vi "Measurement UI.vi"() -> ()   [LabVIEW 2021, in "Ripple_PMIC.lvlib"]
uses:
  Ripple_PMIC.lvlib
panel:
  in  "Tab Control":enum32{"Ripple Voltage", "Hidden Page"}(tab)
  out "OutputVoltageV/STimeGraph":waveform(dbl)(graph) caption="Ripple"
  in  "Source resource name":string caption="SOURCE DEVICE NAME"
  in  "Load resource name":string caption="LOAD DEVICE NAME"
  in  "Scope resource name":string caption="SCOPE DEVICE NAME"
  out "Source voltage":dbl caption="SOURCE VOLTAGE"
  out "Load current":dbl caption="LOAD CURRENT"
  out "RMS ripple voltage":dbl caption="RMS RIPPLE VOLTAGE"
  out "P-P ripple voltage":dbl caption="P-P RIPPLE VOLTAGE"
  out "Source current":dbl caption="SOURCE CURRENT"
  out "Load voltage":dbl caption="LOAD VOLATGE"
  out "Ripple values":dbl[](array[numeric]) caption="RIPPLE VALUES"
  out "dt":dbl caption="DT"
  out "Results":string[][](table) caption="RESULTS"
  in  "Aperture time":dbl=0.005 caption="APERTURE TIME" format="%#_6ps"
  in  "DUT setup time":dbl=0.005 caption="DUT SETUP TIME" format="%#_6ps"
  in  "Measurement configuration":string="Measurement settings"
  out "Status":string
  in  "Scope probe attenuation":dbl=1.0 caption="PROBE ATTENUATION"
  in  "Source configuration":string="Source configuration"
  in  "Scope configuration":string="Scope configuration"
  in  "Load configuration":string="Load configuration"
  in  "Mode of operation":T1(ring)=enum."Perform measurement" caption="MODE OF OPERATION"
  in  "Scope acquisition time":dbl=3.0 caption="ACQUISTION TIME" format="%#_6ps"
  in  "Scope sample rate":dbl=10000.0 caption="SAMPLE RATE" format="%#_6pHz"
  in  "Scope channel name":string="0" caption="CHANNEL NAME"
  in  "ScopeResourceName":refnum<k15> caption="RESOURCE NAME"
  in  "Load voltage limit range":dbl=6.0 caption="VOLTAGE LIMIT RANGE" format="%#_6pV"
  in  "Load current level":dbl=5.0 caption="CURRENT LEVEL" format="%#_6pA"
  in  "ELOADResourceName":refnum<k15> caption="RESOURCE NAME"
  in  "Source current limit":dbl=15.0 caption="CURRENT LIMIT" format="%#_6pA"
  in  "Source voltage level":dbl=10.0 caption="VOLTAGE LEVEL" format="%#_6pV"
  in  "PPSResourceName":refnum<k15> caption="RESOURCE NAME"
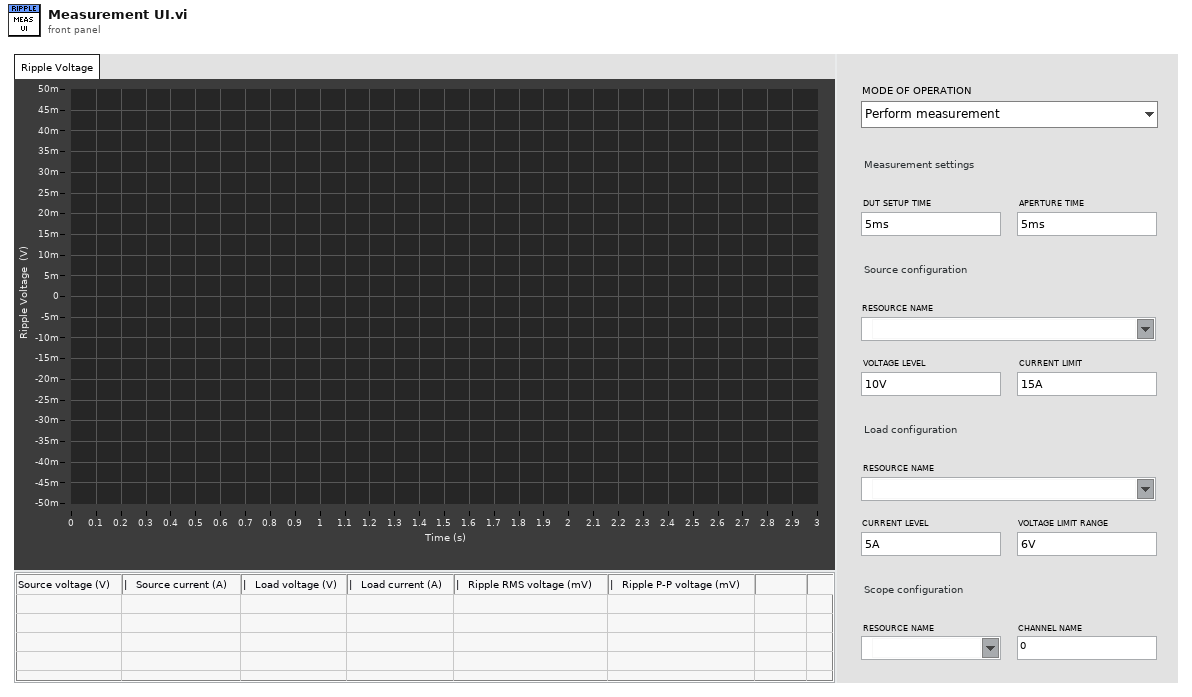
[diagram p1: front panel]
types:
  T1 = enum32{"Power on the DUT", "Perform measurement", "Power off the DUT"}
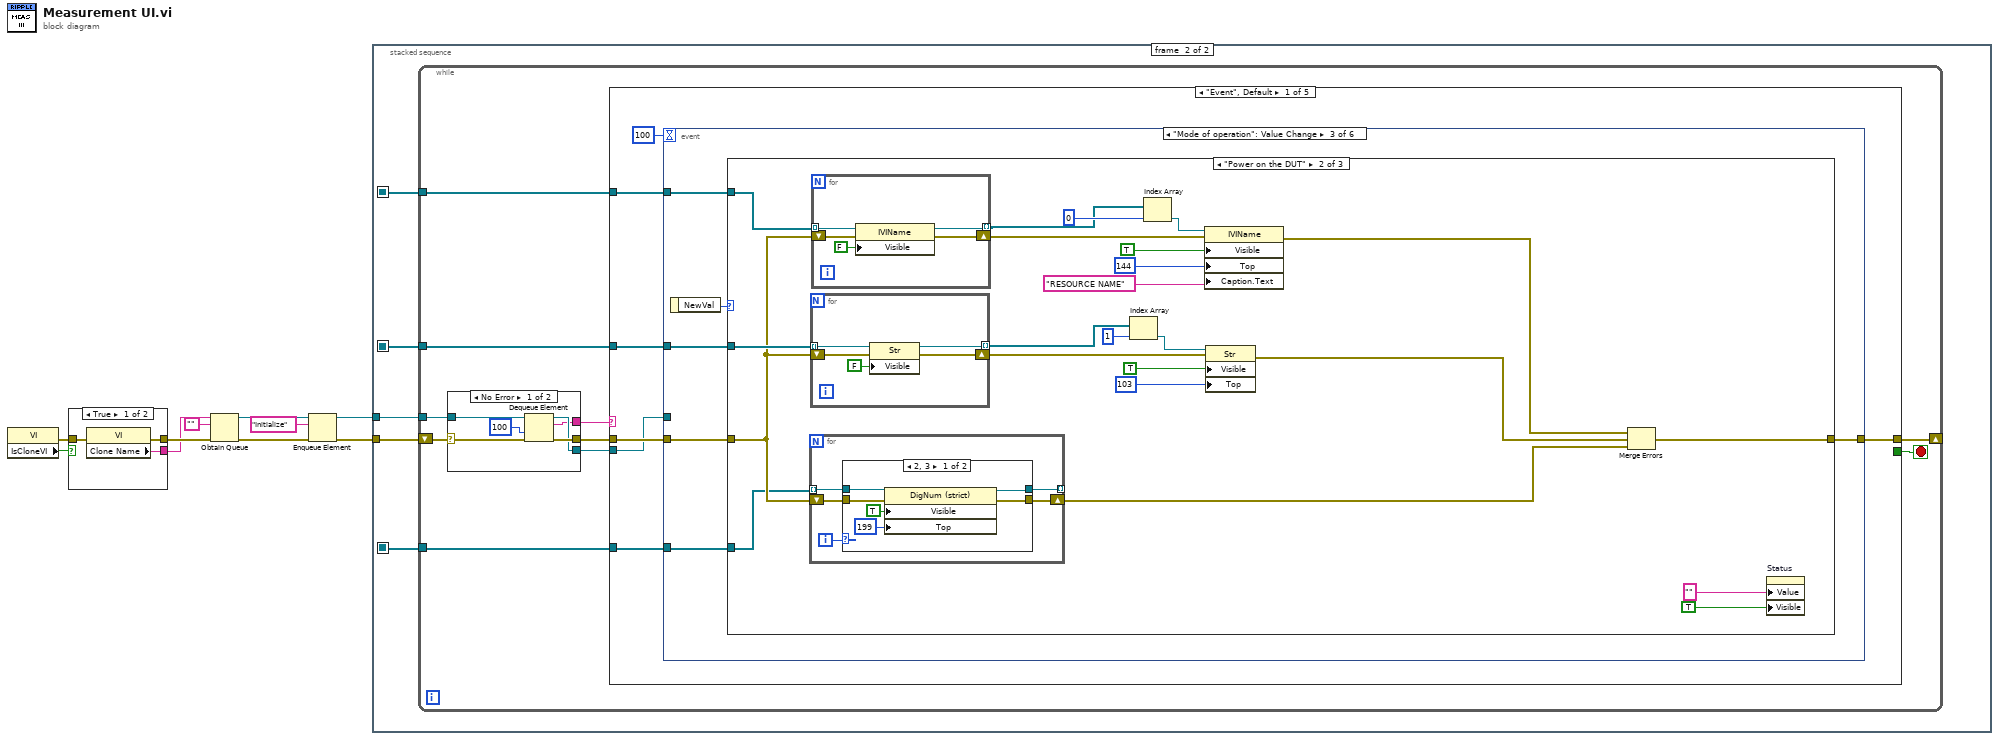
[diagram p0: block diagram]
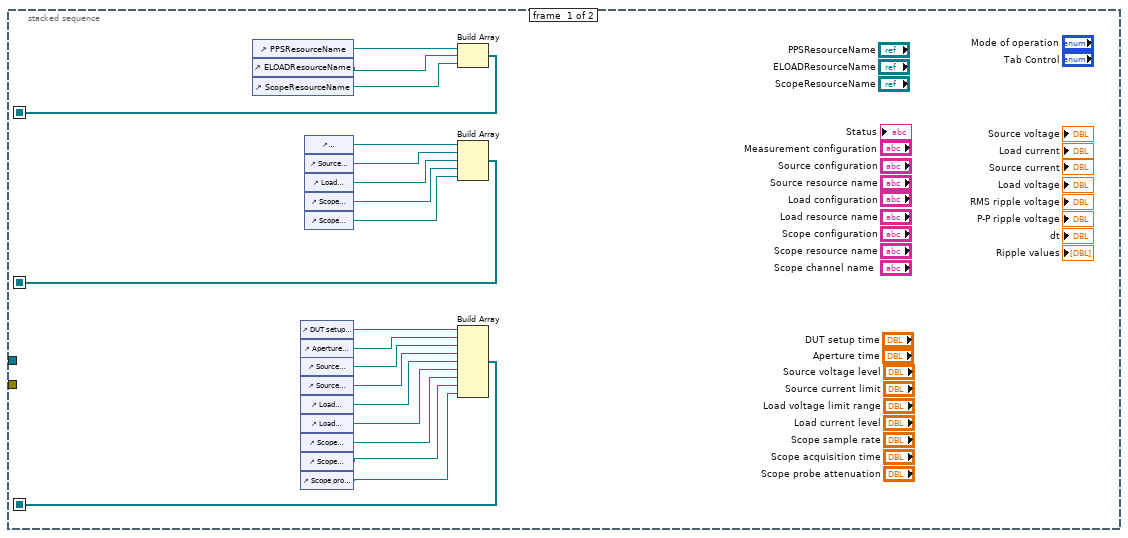
[diagram p2: hidden frame]
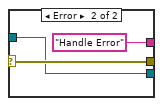
[diagram p3: hidden frame]
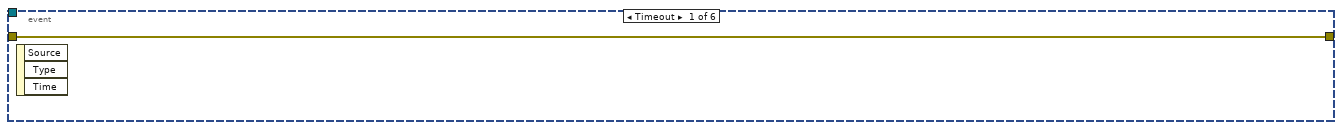
[diagram p4: hidden frame]
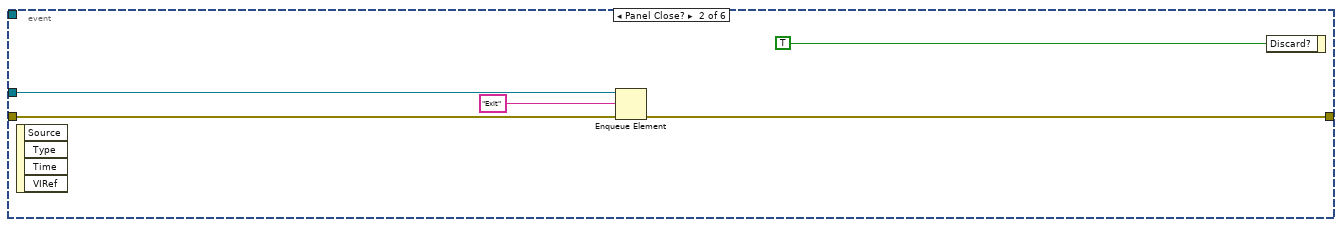
[diagram p5: hidden frame]
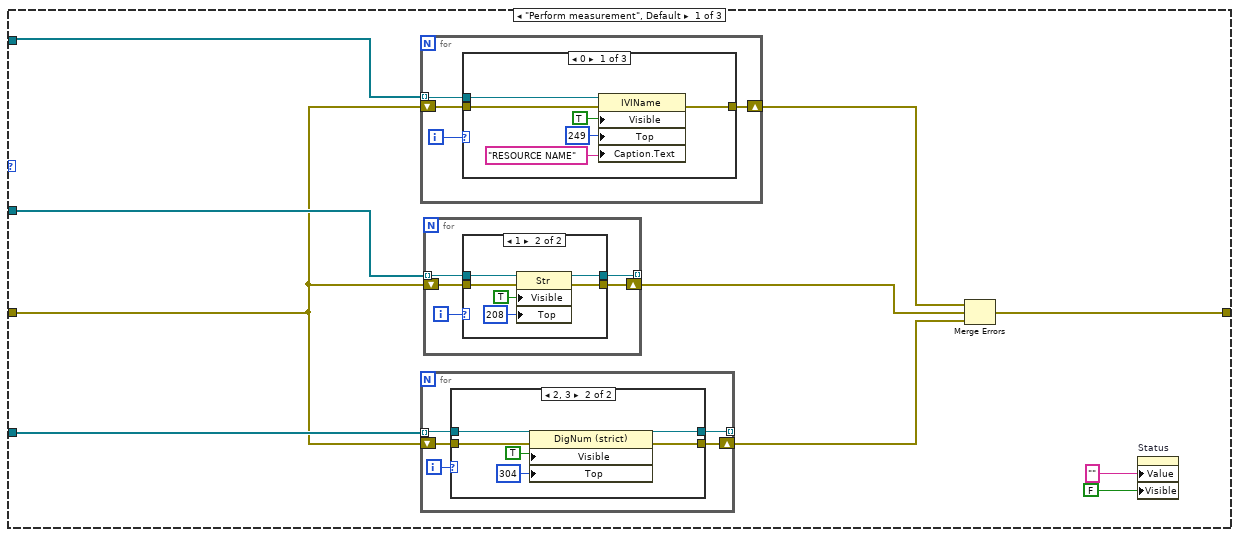
[diagram p6: hidden frame]
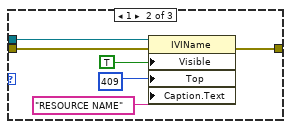
[diagram p7: hidden frame]
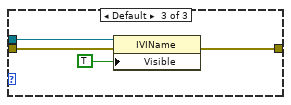
[diagram p8: hidden frame]
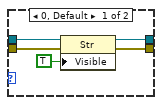
[diagram p9: hidden frame]
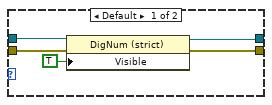
[diagram p10: hidden frame]
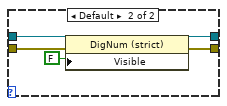
[diagram p11: hidden frame]
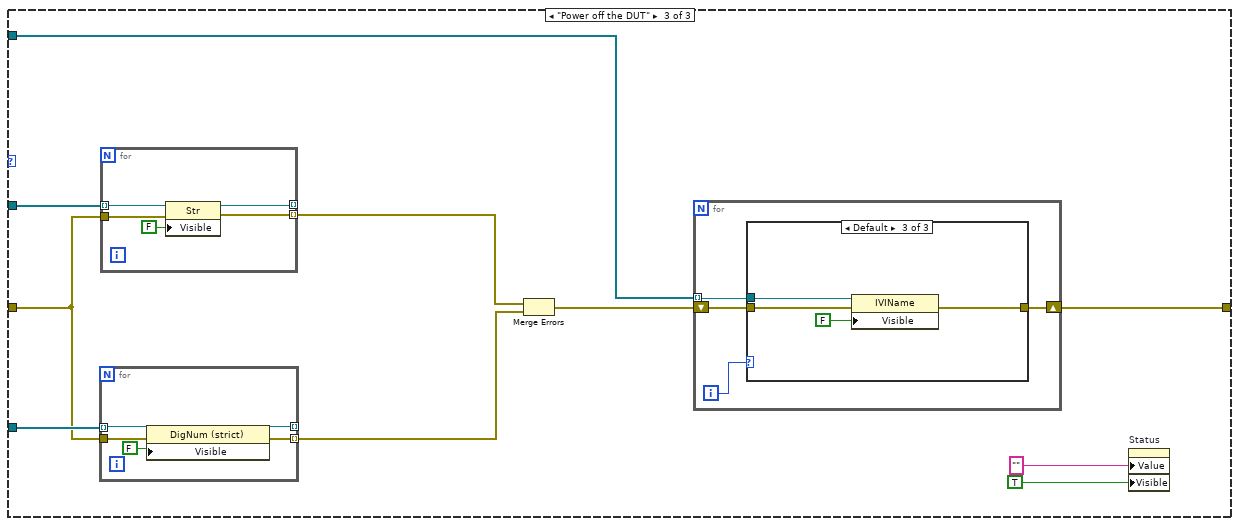
[diagram p12: hidden frame]
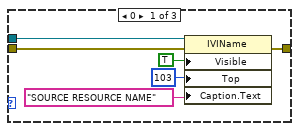
[diagram p13: hidden frame]
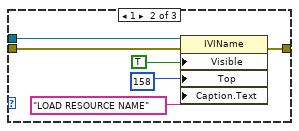
[diagram p14: hidden frame]
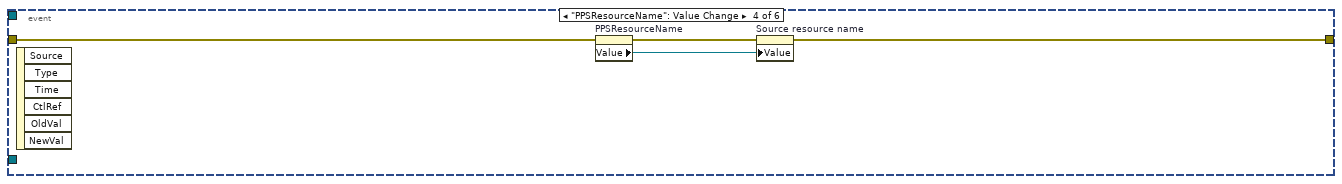
[diagram p15: hidden frame]
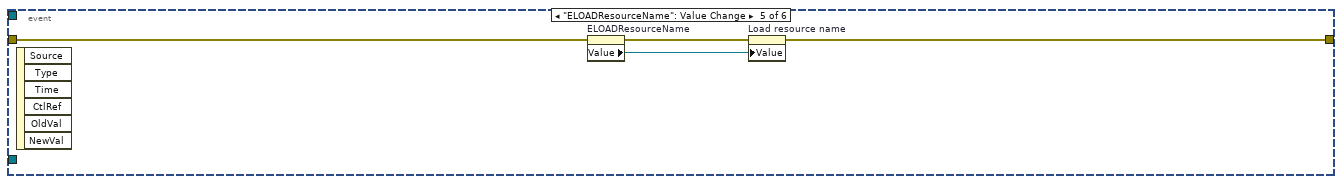
[diagram p16: hidden frame]
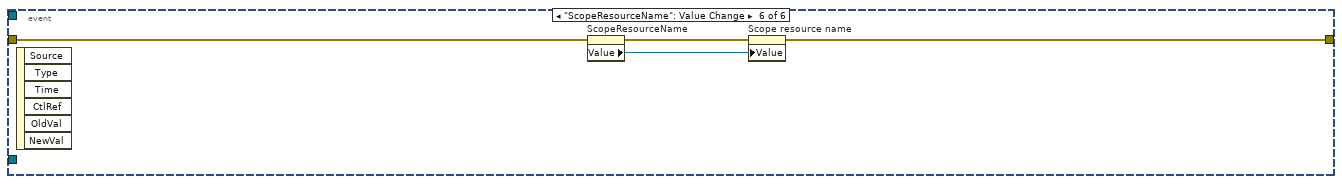
[diagram p17: hidden frame]
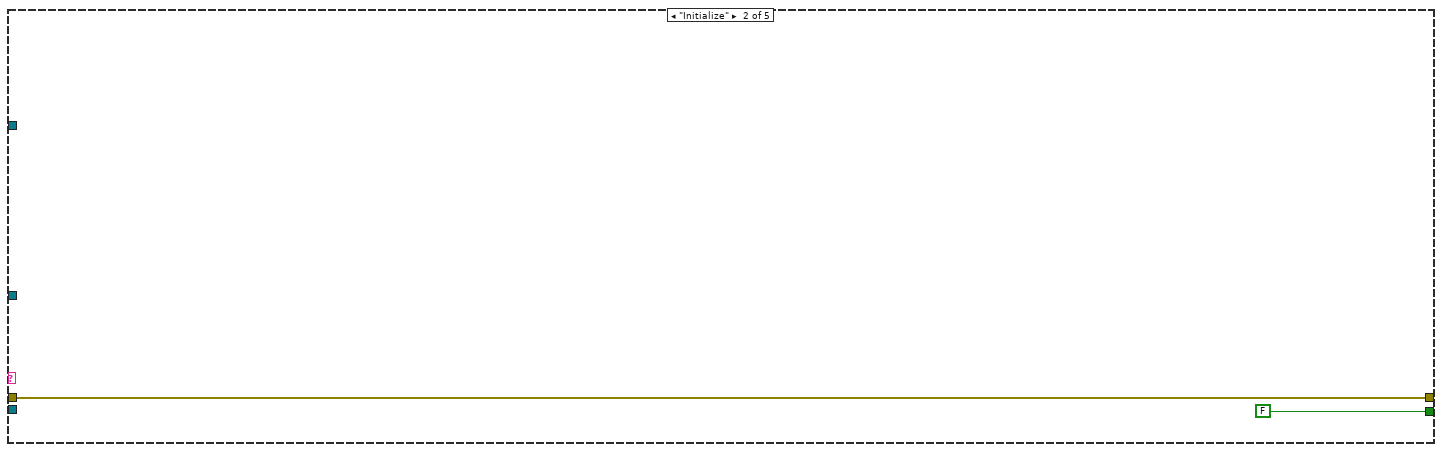
[diagram p18: hidden frame]
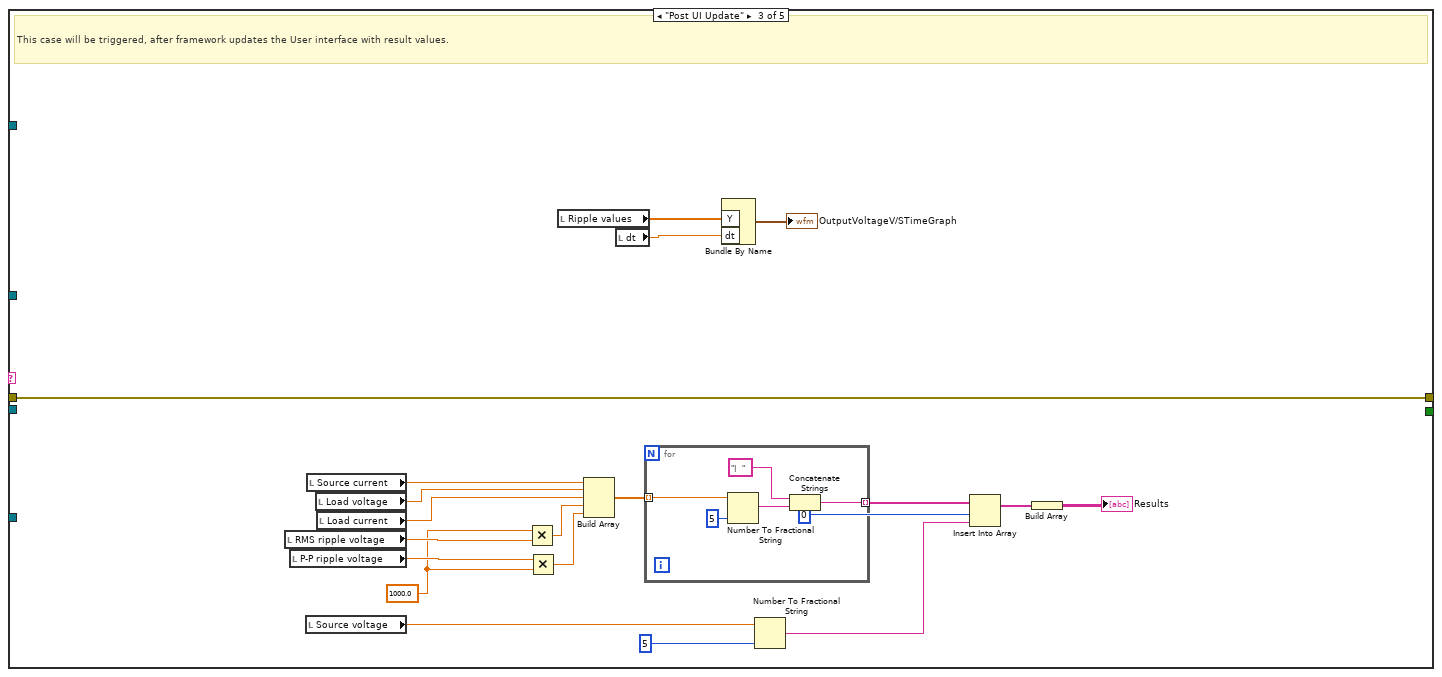
[diagram p19: hidden frame]
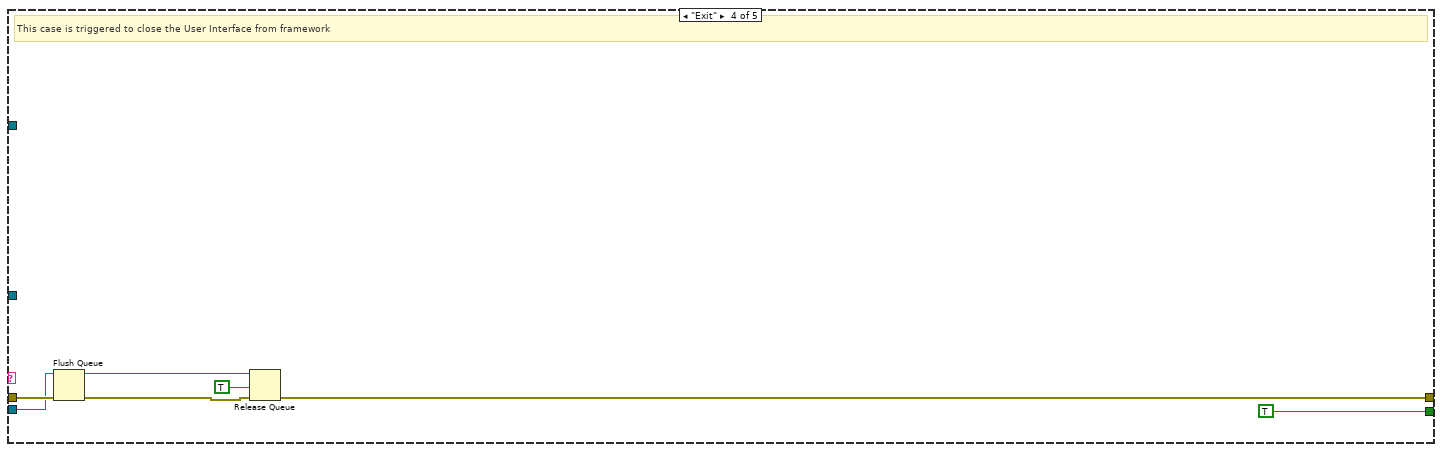
[diagram p20: hidden frame]
diagram:
  n1 = property class="VI"() -> (error out=w1:errorcluster, "IsCloneVI"=w2:bool)  [unwired: 2 in, 1 out]
  n2 = case shown="True" w2 {
    tunnel: [w13 w16] -> w10
    tunnel: [w12 w15] -> w9
    tunnel: w1 -> [w11 w14]
    frame True {
      n3 = property class="VI"(error in=w11) -> (error out=w13:errorcluster, "Clone Name"=w12:string)  [unwired: 1 in, 1 out]
    }
    frame False {
      n4 = property class="VI"(error in=w14) -> (error out=w16:errorcluster, "Name"=w15:string)  [unwired: 1 in, 1 out]
    }
  }
  n5 = Obtain Queue(name (unnamed)=w9, element data type="", error in (no error)=w10) -> (queue out=w6:refnum<queue>, error out=w8:errorcluster)  [unwired: 2 in, 1 out]
  n6 = Enqueue Element(queue=w6, element="Initialize", error in (no error)=w8) -> (queue out=w5:refnum<queue>, error out=w7:errorcluster)  [unwired: 1 in, 1 out]
  n7 = stacked-sequence {
    seq-local: [w25 _] -> [_ w37]
    seq-local: [w24 _] -> [_ w39]
    seq-local: [w23 _] -> [_ w38]
    tunnel: w7 -> [_ w41]
    tunnel: w5 -> [_ w40]
    frame #0 {
      n8 = control-ref of="PPSResourceName"() -> (w28:refnum<vi>)
      n9 = control-ref of="ELOADResourceName"() -> (w27:refnum<vi>)
      n10 = control-ref of="ScopeResourceName"() -> (w26:refnum<vi>)
      n11 = control-ref of="DUT setup time"() -> (w18:refnum<vi>)
      n12 = control-ref of="Aperture time"() -> (w17:refnum<vi>)
      n13 = control-ref of="Source voltage level"() -> (w36:refnum<vi>)
      n14 = control-ref of="Source current limit"() -> (w34:refnum<vi>)
      n15 = control-ref of="Load voltage limit range"() -> (w32:refnum<vi>)
      n16 = control-ref of="Load current level"() -> (w31:refnum<vi>)
      n17 = control-ref of="Scope sample rate"() -> (w30:refnum<vi>)
      n18 = control-ref of="Scope acquisition time"() -> (w33:refnum<vi>)
      n19 = control-ref of="Scope probe attenuation"() -> (w35:refnum<vi>)
      n20 = control-ref of="Measurement configuration"() -> (w19:refnum<vi>)
      n21 = control-ref of="Source configuration"() -> (w29:refnum<vi>)
      n22 = control-ref of="Load configuration"() -> (w22:refnum<vi>)
      n23 = control-ref of="Scope configuration"() -> (w21:refnum<vi>)
      n24 = control-ref of="Scope channel name"() -> (w20:refnum<vi>)
      n25 = Build Array(w28, w27, w26) -> (w25:refnum<vi>[])
      n26 = Build Array(w19, w29, w22, w21, w20) -> (w24:refnum<vi>[])
      n27 = Build Array(w18, w17, w36, w34, w32, w31, w30, w33, w35) -> (w23:refnum<vi>[])
    }
    frame #1 {
      n28 = while {
        shift-right: [w46] -> _
        shift-left: w41 -> [w51]
        tunnel: w40 -> [w49]
        tunnel: w39 -> [w44]
        tunnel: w38 -> [w43]
        tunnel: w37 -> [w42]
        stop <- w45 stop-if-true
        n29 = case shown="No Error" w51 {
          selector: w51 -> [w57 w60]
          tunnel: [w56 w60] -> w50
          tunnel: w49 -> [w55 w59]
          tunnel: [w54 w59] -> w48
          tunnel: [w53 "Handle Error"] -> w47
          frame No Error {
            n30 = Dequeue Element(queue=w55, timeout in ms (-1)=100, error in (no error)=w57) -> (queue out=w54:refnum<queue>, element=w53:string, error out=w56:errorcluster)  [unwired: 1 out]
          }
          frame Error {
          }
        }
        n31 = case shown="\"Event\", Default" w47 {
          tunnel: w50 -> [w66 w243 w250 w276 w277]
          tunnel: w48 -> [w65 _ _ w274 _]
          tunnel: [w67 w243 w250 w271 w277] -> w46
          tunnel: [_ FALSE _ TRUE _] -> w45
          tunnel: w44 -> [w63 _ _ _ _]
          tunnel: w43 -> [w62 _ _ _ _]
          tunnel: w42 -> [w61 _ _ _ _]
          frame "Event", Default {
            n32 = event shown="[2] \"Mode of operation\": Value Change" {
              selector: _ -> [_ _ _ _ _ _]
              dyn-events: _ -> [_ _ _ _ _ _]
              timeout: 100 -> [_ _ _ _ _ _]
              tunnel: [w68 w72 w74 w231 w235 w239] -> w67
              tunnel: w66 -> [w68 w73 w79 w233 w237 w241]
              tunnel: w65 -> [_ w71 _ _ _ _]
              tunnel: w63 -> [_ _ w77 _ _ _]
              tunnel: w62 -> [_ _ w76 _ _ _]
              tunnel: w61 -> [_ _ w75 _ _ _]
              event Timeout {
                n33 = event-data() -> ()  [unwired: 1 in, 3 out]
              }
              event Panel Close? {
                n34 = event-data() -> ()  [unwired: 1 in, 4 out]
                n35 = Enqueue Element(queue=w71, element="Exit", error in (no error)=w73) -> (error out=w72:errorcluster)  [unwired: 1 in, 2 out]
                n36 = event-data("Discard?"=TRUE) -> ()  [unwired: 1 in, 1 out]
              }
              event "Mode of operation": Value Change {
                n37 = event-data() -> ("NewVal"=w78:T1)  [unwired: 1 in]
                n38 = case shown="\"Power on the DUT\"" w78 {
                  tunnel: w79 -> [w84 w157 w198]
                  tunnel: w77 -> [w89 w164 w199]
                  tunnel: w76 -> [w88 w156 w200]
                  tunnel: w75 -> [w87 w158 w197]
                  tunnel: [w83 w146 w193] -> w74
                  frame "Perform measurement", Default {
                    n39 = for {
                      shift-right: [w91] -> w82
                      shift-left: w84 -> [w92]
                      tunnel: w87 -> [w90] mode=indexing
                      i -> [w93]
                      n40 = case shown="0" w93 {
                        tunnel: w92 -> [w96 w102 w109]
                        tunnel: [w95 w101 w107] -> w91
                        tunnel: w90 -> [w94 w100 w106]
                        frame 0 {
                          n41 = property class="IVIName"(reference=w94, error in=w96, "Visible"=TRUE, "Top"=249 ("Position:Top"), "Caption.Text"="RESOURCE NAME") -> (error out=w95:errorcluster)  [unwired: 1 out]
                        }
                        frame 1 {
                          n42 = property class="IVIName"(reference=w100, error in=w102, "Visible"=TRUE, "Top"=409 ("Position:Top"), "Caption.Text"="RESOURCE NAME") -> (error out=w101:errorcluster)  [unwired: 1 out]
                        }
                        frame Default {
                          n43 = property class="IVIName"(reference=w106, error in=w109, "Visible"=TRUE) -> (error out=w107:errorcluster)  [unwired: 1 out]
                        }
                      }
                    }
                    n44 = for {
                      tunnel: w88 -> [w130] mode=indexing
                      tunnel: [w129] -> _ mode=indexing
                      shift-right: [w127] -> w80
                      shift-left: w84 -> [w128]
                      i -> [w126]
                      n45 = case shown="2, 3" w126 {
                        tunnel: w130 -> [w135 w141]
                        tunnel: [w132 w139] -> w129
                        tunnel: w128 -> [w134 w138]
                        tunnel: [w133 w137] -> w127
                        frame Default {
                          n46 = property class="DigNum (strict)"(reference=w135, error in=w134, "Visible"=TRUE) -> (reference out=w132:refnum<vi>, error out=w133:errorcluster)
                        }
                        frame 2, 3 {
                          n47 = property class="DigNum (strict)"(reference=w141, error in=w138, "Visible"=TRUE, "Top"=304 ("Position:Top")) -> (reference out=w139:refnum<vi>, error out=w137:errorcluster)
                        }
                      }
                    }
                    n48 = for {
                      tunnel: w89 -> [w114] mode=indexing
                      tunnel: [w112] -> _ mode=indexing
                      shift-right: [w111] -> w81
                      shift-left: w84 -> [w113]
                      i -> [w110]
                      n49 = case shown="1" w110 {
                        tunnel: w114 -> [w118 w124]
                        tunnel: w113 -> [w115 w123]
                        tunnel: [w117 w122] -> w112
                        tunnel: [w116 w121] -> w111
                        frame 0, Default {
                          n50 = property class="Str"(reference=w118, error in=w115, "Visible"=TRUE) -> (reference out=w117:refnum<vi>, error out=w116:errorcluster)
                        }
                        frame 1 {
                          n51 = property class="Str"(reference=w124, error in=w123, "Visible"=TRUE, "Top"=208 ("Position:Top")) -> (reference out=w122:refnum<vi>, error out=w121:errorcluster)
                        }
                      }
                    }
                    n52 = Merge Errors(w82, w81, w80) -> (w83:errorcluster)
                    n53 = property on="Status" class="Str"("Value"="" ("Status"), "Visible"=FALSE) -> ()  [unwired: 2 in, 2 out]
                  }
                  frame "Power on the DUT" {
                    n54 = for {
                      tunnel: w156 -> [w179] mode=indexing
                      tunnel: [w178] -> _ mode=indexing
                      shift-right: [w176] -> w142
                      shift-left: w157 -> [w177]
                      i -> [w175]
                      n55 = case shown="2, 3" w175 {
                        tunnel: w179 -> [w183 w190]
                        tunnel: [w185 w188] -> w178
                        tunnel: w177 -> [w182 w187]
                        tunnel: [w184 w186] -> w176
                        frame 2, 3 {
                          n56 = property class="DigNum (strict)"(reference=w183, error in=w182, "Visible"=TRUE, "Top"=199 ("Position:Top")) -> (reference out=w185:refnum<vi>, error out=w184:errorcluster)
                        }
                        frame Default {
                          n57 = property class="DigNum (strict)"(reference=w190, error in=w187, "Visible"=FALSE) -> (reference out=w188:refnum<vi>, error out=w186:errorcluster)
                        }
                      }
                    }
                    n58 = for {
                      tunnel: w164 -> [w173] mode=indexing
                      tunnel: [w171] -> w160 mode=indexing
                      shift-right: [w170] -> w161
                      shift-left: w157 -> [w172]
                      n59 = property class="Str"(reference=w173, error in=w172, "Visible"=FALSE) -> (reference out=w171:refnum<vi>, error out=w170:errorcluster)
                    }
                    n60 = for {
                      tunnel: w158 -> [w168] mode=indexing
                      tunnel: [w166] -> w151 mode=indexing
                      shift-right: [w165] -> w152
                      shift-left: w157 -> [w167]
                      n61 = property class="IVIName"(reference=w168, error in=w167, "Visible"=FALSE) -> (reference out=w166:refnum<vi>, error out=w165:errorcluster)
                    }
                    n62 = Index Array(array=w160, index=1) -> (element=w159:refnum<vi>)
                    n63 = Index Array(array=w151, index=0) -> (element=w153:refnum<vi>)
                    n64 = property class="IVIName"(reference=w153, error in=w152, "Visible"=TRUE, "Top"=144 ("Position:Top"), "Caption.Text"="RESOURCE NAME") -> (error out=w147:errorcluster)  [unwired: 1 out]
                    n65 = property class="Str"(reference=w159, error in=w161, "Visible"=TRUE, "Top"=103 ("Position:Top")) -> (error out=w148:errorcluster)  [unwired: 1 out]
                    n66 = Merge Errors(w147, w148, w142) -> (w146:errorcluster)
                    n67 = property on="Status" class="Str"("Value"="" ("Status"), "Visible"=TRUE) -> ()  [unwired: 2 in, 2 out]
                  }
                  frame "Power off the DUT" {
                    n68 = for {
                      tunnel: w200 -> [w230] mode=indexing
                      tunnel: [w228] -> _ mode=indexing
                      tunnel: w198 -> [w227]
                      tunnel: [w226] -> w195 mode=indexing
                      n69 = property class="DigNum (strict)"(reference=w230, error in=w227, "Visible"=FALSE) -> (reference out=w228:refnum<vi>, error out=w226:errorcluster)
                    }
                    n70 = for {
                      tunnel: w199 -> [w224] mode=indexing
                      tunnel: w198 -> [w223]
                      tunnel: [w222] -> _ mode=indexing
                      tunnel: [w221] -> w196 mode=indexing
                      n71 = property class="Str"(reference=w224, error in=w223, "Visible"=FALSE) -> (reference out=w222:refnum<vi>, error out=w221:errorcluster)
                    }
                    n72 = Merge Errors(w196, w195) -> (w194:errorcluster)
                    n73 = for {
                      tunnel: w197 -> [w203] mode=indexing
                      shift-right: [w201] -> w193
                      shift-left: w194 -> [w202]
                      i -> [w204]
                      n74 = case shown="Default" w204 {
                        tunnel: w203 -> [w207 w212 w220]
                        tunnel: w202 -> [w206 w213 w219]
                        tunnel: [w205 w211 w217] -> w201
                        frame 0 {
                          n75 = property class="IVIName"(reference=w207, error in=w206, "Visible"=TRUE, "Top"=103 ("Position:Top"), "Caption.Text"="SOURCE RESOURCE NAME") -> (error out=w205:errorcluster)  [unwired: 1 out]
                        }
                        frame 1 {
                          n76 = property class="IVIName"(reference=w212, error in=w213, "Visible"=TRUE, "Top"=158 ("Position:Top"), "Caption.Text"="LOAD RESOURCE NAME") -> (error out=w211:errorcluster)  [unwired: 1 out]
                        }
                        frame Default {
                          n77 = property class="IVIName"(reference=w220, error in=w219, "Visible"=FALSE) -> (error out=w217:errorcluster)  [unwired: 1 out]
                        }
                      }
                    }
                    n78 = property on="Status" class="Str"("Value"="" ("Status"), "Visible"=TRUE) -> ()  [unwired: 2 in, 2 out]
                  }
                }
              }
              event "PPSResourceName": Value Change {
                n79 = event-data() -> ()  [unwired: 1 in, 6 out]
                n80 = property on="PPSResourceName" class="IVIName"(error in=w233) -> (error out=w232:errorcluster, "Value"=w234:refnum<k15>)  [unwired: 1 in, 1 out]
                n81 = property on="Source resource name" class="Str"(error in=w232, "Value"=w234) -> (error out=w231:errorcluster)  [unwired: 1 in, 1 out]
              }
              event "ELOADResourceName": Value Change {
                n82 = event-data() -> ()  [unwired: 1 in, 6 out]
                n83 = property on="ELOADResourceName" class="IVIName"(error in=w237) -> (error out=w236:errorcluster, "Value"=w238:refnum<k15>)  [unwired: 1 in, 1 out]
                n84 = property on="Load resource name" class="Str"(error in=w236, "Value"=w238) -> (error out=w235:errorcluster)  [unwired: 1 in, 1 out]
              }
              event "ScopeResourceName": Value Change {
                n85 = event-data() -> ()  [unwired: 1 in, 6 out]
                n86 = property on="ScopeResourceName" class="IVIName"(error in=w241) -> (error out=w240:errorcluster, "Value"=w242:refnum<k15>)  [unwired: 1 in, 1 out]
                n87 = property on="Scope resource name" class="Str"(error in=w240, "Value"=w242) -> (error out=w239:errorcluster)  [unwired: 1 in, 1 out]
              }
            }
          }
          frame "Initialize" {
          }
          frame "Post UI Update" {
            w247 = 1000.0 ("x")
            # "This case will be triggered, after framework updates the User interface with result values."
            n88 = local read "RMS ripple voltage"() -> (w248:dbl)
            n89 = local read "P-P ripple voltage"() -> (w249:dbl)
            n90 = local read "Source voltage"() -> (w256:dbl)
            n91 = local read "Source current"() -> (w261:dbl)
            n92 = local read "Load voltage"() -> (w260:dbl)
            n93 = local read "Load current"() -> (w259:dbl)
            n94 = Multiply(x=w247, y=w248) -> (x*y=w246:dbl)
            n95 = Multiply(x=w249, y=w247) -> (x*y=w245:dbl)
            n96 = local read "Ripple values"() -> (w264:dbl[])
            n97 = Build Array(w261, w260, w259, w246, w245) -> (w258:dbl[])
            n98 = local read "dt"() -> (w263:dbl)
            n99 = for {
              tunnel: w258 -> [w268] mode=indexing
              tunnel: [w265] -> w255 mode=indexing
              n100 = Number To Fractional String(number=w268, precision (6)=i16 5) -> (F-format string=w267:string)  [unwired: 2 in]
              n101 = Concatenate Strings("|   " ("string"), w267) -> (w265:string)
            }
            n102 = Bundle By Name("Y"=w264, "dt"=w263) -> (→"OutputVoltageV/STimeGraph":waveform(dbl))  [unwired: 1 in]
            n103 = Number To Fractional String(number=w256, precision (6)=i16 5) -> (F-format string=w254:string)  [unwired: 2 in]
            n104 = Insert Into Array(array=w255, index=0, new element=w254) -> (w252:string[])
            n105 = Build Array(w252) -> (→"Results":string[][])
          }
          frame "Exit" {
            # "This case is triggered to close the User Interface from framework"
            n106 = Flush Queue(queue=w274, error in (no error)=w276) -> (queue out=w273:refnum<queue>, error out=w272:errorcluster)  [unwired: 1 out]
            n107 = Release Queue(queue=w273, force destroy? (F)=TRUE, error in (no error)=w272) -> (error out=w271:errorcluster)  [unwired: 2 out]
          }
          frame "Handle Error" {
          }
        }
      }
    }
  }
